vi "read_relay.vi"(1 "Relay":i32=1 min=1 max=12, 2 "Slot":i32=10 min=0 max=14) -> (0 "Relay Status":bool)   [LabVIEW 2011]
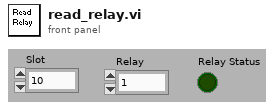
[diagram p1: front panel]
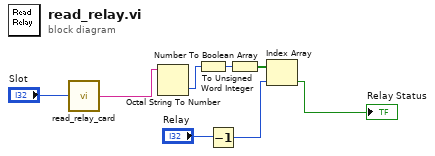
[diagram p0: block diagram]
diagram:
  n1 = call "read_relay_card.vi"("Slot"="Slot") -> ("data"=w2:string)
  n2 = Octal String To Number(4:w2) -> (0:w5:u32)  [unwired: 3 out]
  n3 = To Unsigned Word Integer(number=w5) -> (unsigned 16bit integer=w6:u16)
  n4 = Decrement(x="Relay") -> (x-1=w3:i32)
  n5 = Number To Boolean Array(number=w6) -> (Boolean array=w7:bool[])
  n6 = Index Array(array=w7, index=w3) -> (element=→"Relay Status":bool)
